vi "Mouse Move.vi"(7 "Map Model in":refnum<class "Map Model.lvclass">, 8 "error in (no error)":errorcluster, 10 "Position":T1, 11 "Rectangle Select in":refnum<class "Rectangle Select.lvclass">) -> (0 "error out":errorcluster, 3 "Rectangle Select out":refnum<class "Rectangle Select.lvclass">, 5 "Map Model out":refnum<class "Map Model.lvclass">)   [LabVIEW 2020, in "Map Model.lvlib" / "Rectangle Select.lvclass"]
uses:
  Rectangle Select.lvclass
  E:/Project/Labview-Projects/Completed projects/Map Editor/Models/Map Model/Tools/Tool/Tool.lvclass
  <vilib>/Utility/miscctls.llb/LVPoint32TypeDef.ctl
  Map Model/Map Model.lvclass
  Tool/Tool.lvclass/Tool.ctl
  Map Model/Map Model.lvclass/Map Model.ctl
  Tool/Tool.lvclass
panel:
  # "NOTICE -- YOU MUST LEAVE THIS NOTICE IN PLACE.\n\nCopyright (c) 2017, LIANG LIU Shawn.Liu.cn@gmail.com\nAll rights reserved.\n\nRedistribution and use in source and binary forms, with or without modification, are permitted provided that the following conditions are met:\n-Redistributions of source code must retain the above copyright notice, this list of conditions and the following disclaimer.\n-Redistributions in binary form must reproduce the above copyright notice, this list of conditions and the following disclaimer in the documentation and/or other materials provided with the distribution.\n-Neither the name of the eLp nor the names of its contributors may be used to endorse or promote products derived from this software without specific prior written permission.\n\nTHIS SOFTWARE IS PROVIDED BY THE COPYRIGHT HOLDERS AND CONTRIBUTORS \"AS IS\" AND ANY EXPRESS OR IMPLIED WARRANTIES, INCLUDING, BUT NOT LIMITED TO, THE IMPLIED WARRANTIES OF MERCHANTABILITY AND FITNESS FOR A PARTICULAR PURPOSE ARE DISCLAIMED. IN NO EVENT SHALL THE COPYRIGHT HOLDER OR CONTRIBUTORS BE LIABLE FOR ANY DIRECT, INDIRECT, INCIDENTAL, SPECIAL, EXEMPLARY, OR CONSEQUENTIAL DAMAGES (INCLUDING, BUT NOT LIMITED TO, PROCUREMENT OF SUBSTITUTE GOODS OR SERVICES; LOSS OF USE, DATA, OR PROFITS; OR BUSINESS INTERRUPTION) HOWEVER CAUSED AND ON ANY THEORY OF LIABILITY, WHETHER IN CONTRACT, STRICT LIABILITY, OR TORT (INCLUDING NEGLIGENCE OR OTHERWISE) ARISING IN ANY WAY OUT OF THE USE OF THIS SOFTWARE, EVEN IF ADVISED OF THE POSSIBILITY OF SUCH DAMAGE."
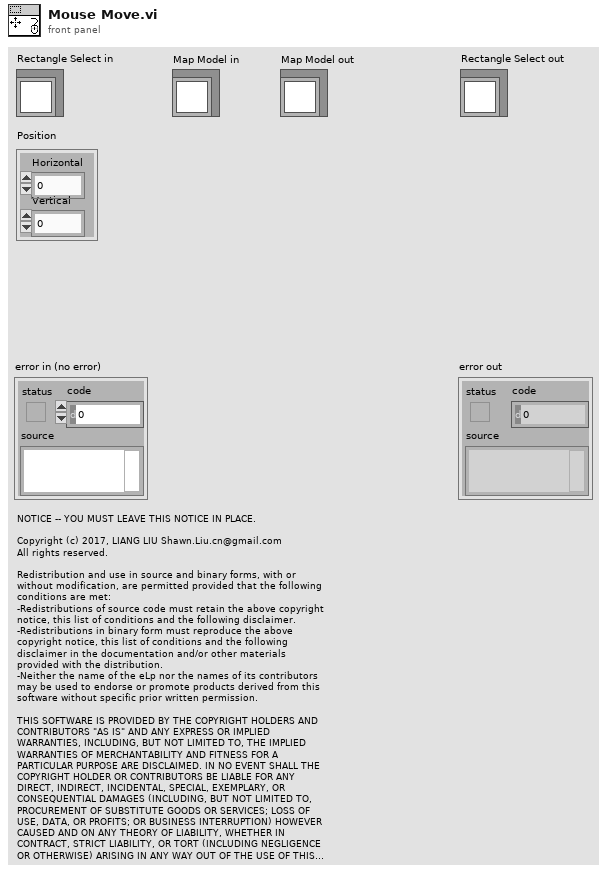
[diagram p1: front panel]
types:
  T1 = typedef "LVPoint32TypeDef.ctl" = cluster{"Horizontal":i32, "Vertical":i32}
  T2 = cluster{"Width":i16, "Style":enum32{"Solid", "Dash", "Dot", "DashDot", "DashDotDot"}}
  T3 = cluster{"Occupied Color":cluster{"Value":u8, "Color":u32}, "Free Color":cluster{"Value":u8, "Color":u32}, "Unknown Color":cluster{"Value":u8, "Color":u32}}
  T4 = cluster{"left":i16, "top":i16, "right":i16, "bottom":i16}
  T5 = typedef "LVPointTypeDef.ctl" = cluster{"Horizontal":i16, "Vertical":i16}
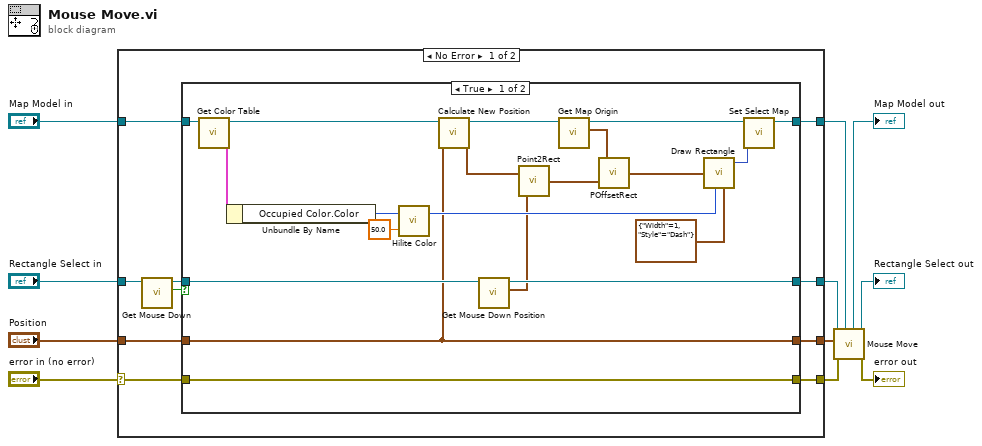
[diagram p0: block diagram]
diagram:
  n1 = case shown="No Error" "error in (no error)" {
    selector: "error in (no error)" -> [w14 w49]
    tunnel: [w21 w46] -> w11
    tunnel: [w20 w49] -> w10
    tunnel: [w19 w48] -> w9
    tunnel: [w18 w47] -> w8
    tunnel: "Map Model in" -> [w17 w48]
    tunnel: "Rectangle Select in" -> [w16 w47]
    tunnel: "Position" -> [w15 w46]
    frame No Error {
      n2 = call "Get Mouse Down.vi"("Tool in"=w16) -> ("Mouse Down"=w12:bool, "Tool out"=w13:refnum<class "Rectangle Select.lvclass">)  [unwired: 9 in]
      n3 = case shown="True" w12 {
        tunnel: w13 -> [w41 w45]
        tunnel: w17 -> [w40 w42]
        tunnel: [w22 w42] -> w19
        tunnel: [w39 w45] -> w18
        tunnel: w15 -> [w29 w43]
        tunnel: [w29 w43] -> w21
        tunnel: w14 -> [w33 w44]
        tunnel: [w33 w44] -> w20
        frame True {
          n4 = call "Get Color Table.vi"("Map Model in"=w40) -> ("Color Table"=w35:T3, "Map Model out"=w36:refnum<class "Map Model.lvclass">)  [unwired: 9 in]
          n5 = Unbundle By Name(w35) -> ("Occupied Color.Color"=w34:u32)
          n6 = call <vilib>:"Hilite Color.vi"("Percentage(30)"=50.0, "Color In"=w34) -> ("Hilite"=w32:u32)  [unwired: 1 out]
          n7 = call "Calculate New Position.vi"("Position in"=w29, "Map Model in"=w36) -> ("Position out"=w27:T1, "Map Model out"=w30:refnum<class "Map Model.lvclass">)  [unwired: 8 in]
          n8 = call "Get Mouse Down Position.vi"("Tool in"=w41) -> ("Mouse Down Position"=w26:T1, "Tool out"=w39:refnum<class "Rectangle Select.lvclass">)  [unwired: 9 in]
          n9 = call <vilib>:"Point2Rect.vi"("point b"=w26, "point a"=w27) -> ("rect"=w23:T4)
          n10 = call "Get Map Origin.vi"("Map Model in"=w30) -> ("Map Origin"=w25:T5, "Map Model out"=w37:refnum<class "Map Model.lvclass">)  [unwired: 9 in]
          n11 = call <vilib>:"POffsetRect.vi"("rect"=w23, "point"=w25) -> ("offset rect"=w24:T4)
          n12 = call <vilib>:"Draw Rectangle.vi"("rect"=w24, "color(black)"=w32, "pen"=T2 {"Width"=1, "Style"=enum."Dash"}) -> ("new picture"=w38:picture)  [unwired: 6 in]
          n13 = call "Set Select Map.vi"("Select Map"=w38, "Map Model in"=w37) -> ("Map Model out"=w22:refnum<class "Map Model.lvclass">)  [unwired: 9 in]
        }
        frame False {
        }
      }
    }
    frame Error {
    }
  }
  n14 = call-parent "Mouse Move.vi"("Map Model in"=w9, "error in (no error)"=w10, "Position"=w11, "Tool in"=w8) -> ("error out"=→"error out":errorcluster, "Tool out"=→"Rectangle Select out":refnum<class "Rectangle Select.lvclass">, "Map Model out"=→"Map Model out":refnum<class "Map Model.lvclass">)  [unwired: 5 in]
